vi "Init.vi"(8 "error in (no error)":errorcluster, 11 "URLPattern in":refnum<class "URLPattern.lvclass">) -> (0 "error out":errorcluster, 3 "URLPattern out":refnum<class "URLPattern.lvclass">)   [LabVIEW 2020, in "Stream.lvlib" / "URLPattern.lvclass"]
uses:
  URLPattern.lvclass
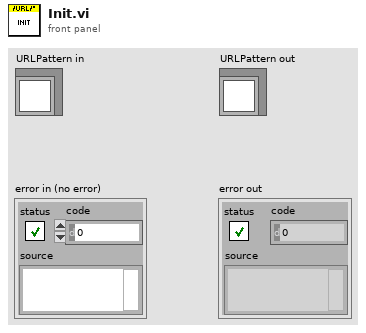
[diagram p1: front panel]
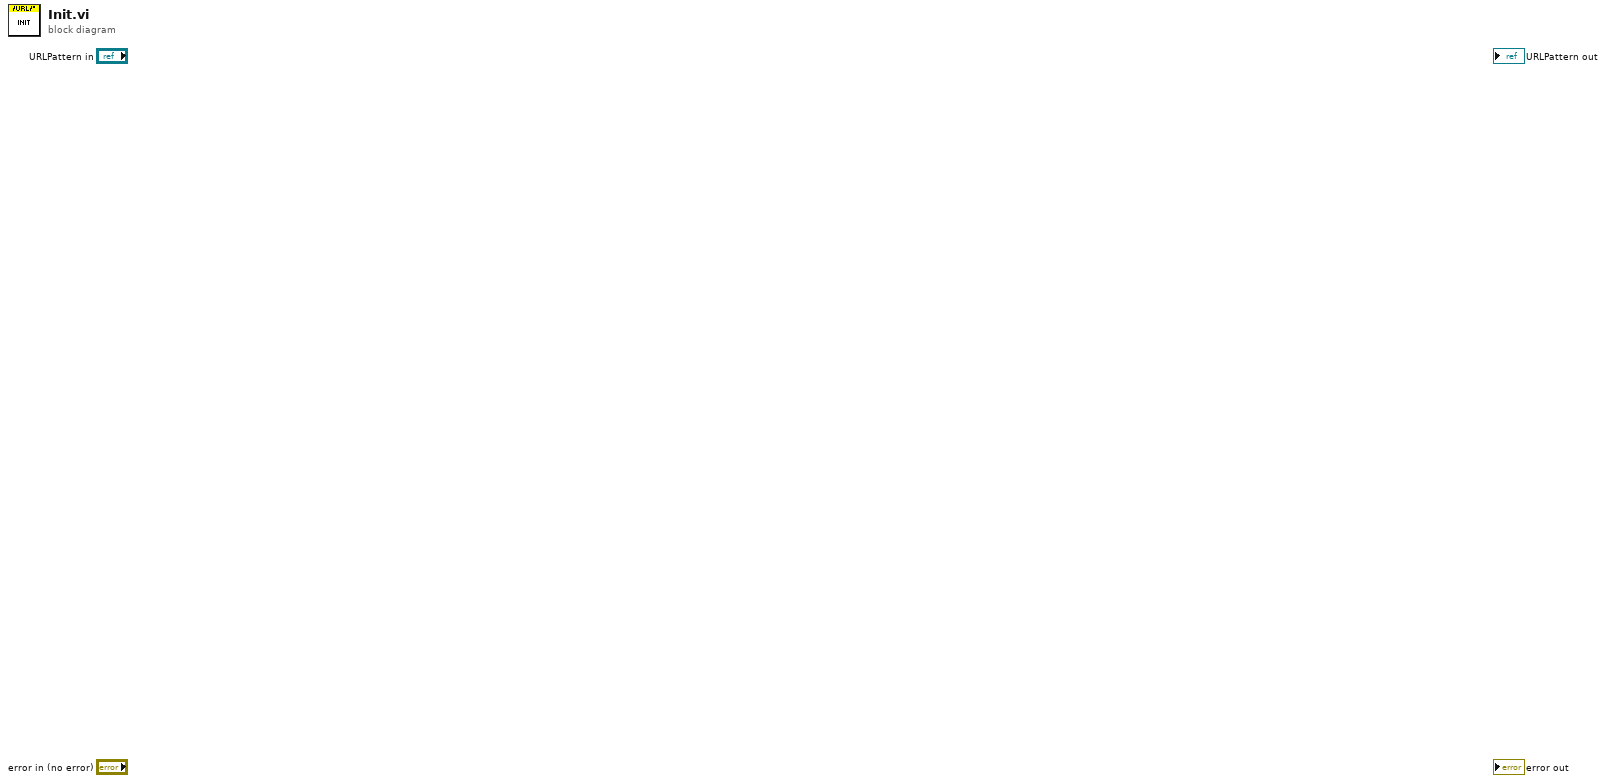
[diagram p0: block diagram]
diagram:
